vi "drive diraction.vi"() -> ()   [LabVIEW 2016]
panel:
  in  "drive diraction":bool
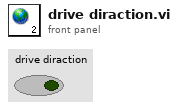
[diagram p1: front panel]
diagram:
